vi "FileIO-Get Preset Parameter File.vi"(0 "Presets":refnum<vi>, 7 "folder":path) -> (4 "Name":string, 8 "selected":path)   [LabVIEW 2020]
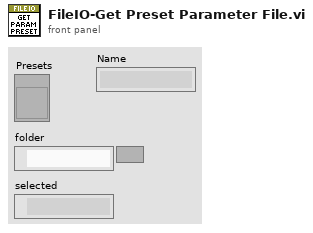
[diagram p1: front panel]
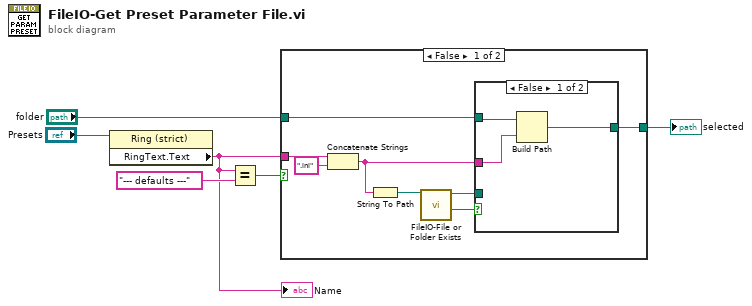
[diagram p0: block diagram]
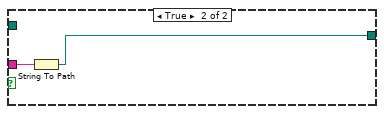
[diagram p3: hidden frame]
diagram:
  n1 = property on="Property Node" class="Ring (strict)"(reference="Presets") -> ("RingText.Text"=w4:string)  [unwired: 1 in, 2 out]
  "Name" <- w4
  n2 = Equal?(x=w4, y="--- defaults ---") -> (x = y?=w5:bool)
  n3 = case shown="False" w5 {
    tunnel: w4 -> [w14 w20]
    tunnel: [w10 w19] -> w2
    tunnel: "folder" -> [w8 _]
    frame False {
      n4 = Concatenate Strings(w14, ".ini" ("string")) -> (w7:string)
      n5 = String To Path(string=w7) -> (path=w12:path)
      n6 = call "FileIO-File or Folder Exists.vi"("path"=w12) -> ("Exists?"=w11:bool, "dup path"=w9:path)  [unwired: 7 in, 2 out]
      n7 = case shown="False" w11 {
        tunnel: [w15 w18] -> w10
        tunnel: w9 -> [_ w18]
        tunnel: w8 -> [w17 _]
        tunnel: w7 -> [w16 _]
        frame False {
          n8 = Build Path(base path=w17, name or relative path=w16) -> (appended path=w15:path)
        }
        frame True {
        }
      }
    }
    frame True {
      n9 = String To Path(string=w20) -> (path=w19:path)
    }
  }
  "selected" <- w2
